vi "Binary_write.vi"(8 "data":cluster{}) -> ()   [LabVIEW 2015]
uses:
  Robot Global Data.vi
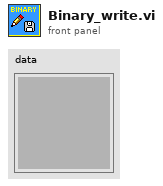
[diagram p1: front panel]
types:
  T1 = enum16{"open", "replace", "create", "open or create", "replace or create", "replace or create with confirmation"}
  T2 = cluster{"Record?":bool, "Current File":string, "Run script?":bool, "Stop recording?":bool, "Stop script?":bool}
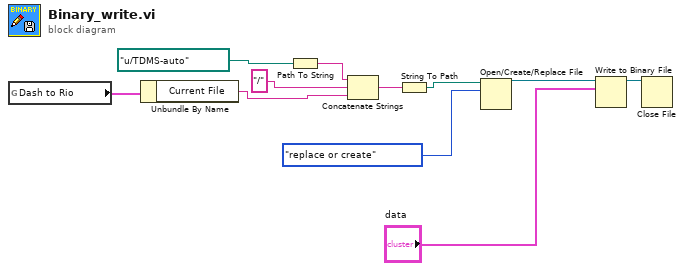
[diagram p0: block diagram]
diagram:
  n1 = global read "Robot Global Data.vi" "Dash to Rio"() -> (w8:T2)
  n2 = Unbundle By Name(w8) -> ("Current File"=w7:string)
  n3 = Path To String(path=path "u:/TDMS-auto" ("file path 3")) -> (string=w11:string)
  n4 = Concatenate Strings(w11, "/" ("TDMS file name"), w7) -> (w9:string)
  n5 = String To Path(string=w9) -> (path=w5:path)
  n6 = Open/Create/Replace File(file path (use dialog)=w5, operation (0:open)=T1."replace or create") -> (refnum out=w3:refnum<file>)  [unwired: 4 in, 2 out]
  n7 = Write to Binary File(file (use dialog)=w3, data="data") -> (refnum out=w1:refnum<file>)  [unwired: 4 in, 2 out]
  n8 = Close File(refnum=w1) -> ()  [unwired: 1 in, 2 out]
